vi "TCPIP_main.vi"() -> ()   [LabVIEW 2018]
uses:
  <vilib>/Utility/error.llb/DialogType.ctl
  TCPIP_main_global.vi
panel:
  in  "Write+Read 2":bool
  out "data out":string
  in  "stop":bool
  in  "Write+Read":bool
  in  "Write":bool
  # "Please run python first\n.exe or .py\npython is server"
  # "This is a template for\nsomeone who don't\nuse pythonnode or \nhave trouble to install \ntensorflow, you can \ntrigger python by tcpip"
  # "Rikcy"
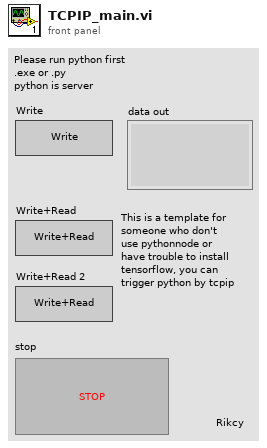
[diagram p1: front panel]
types:
  T1 = typedef "DialogType.ctl" = u16
  T2 = enum16{"Standard", "Buffered", "CRLF", "Immediate"}
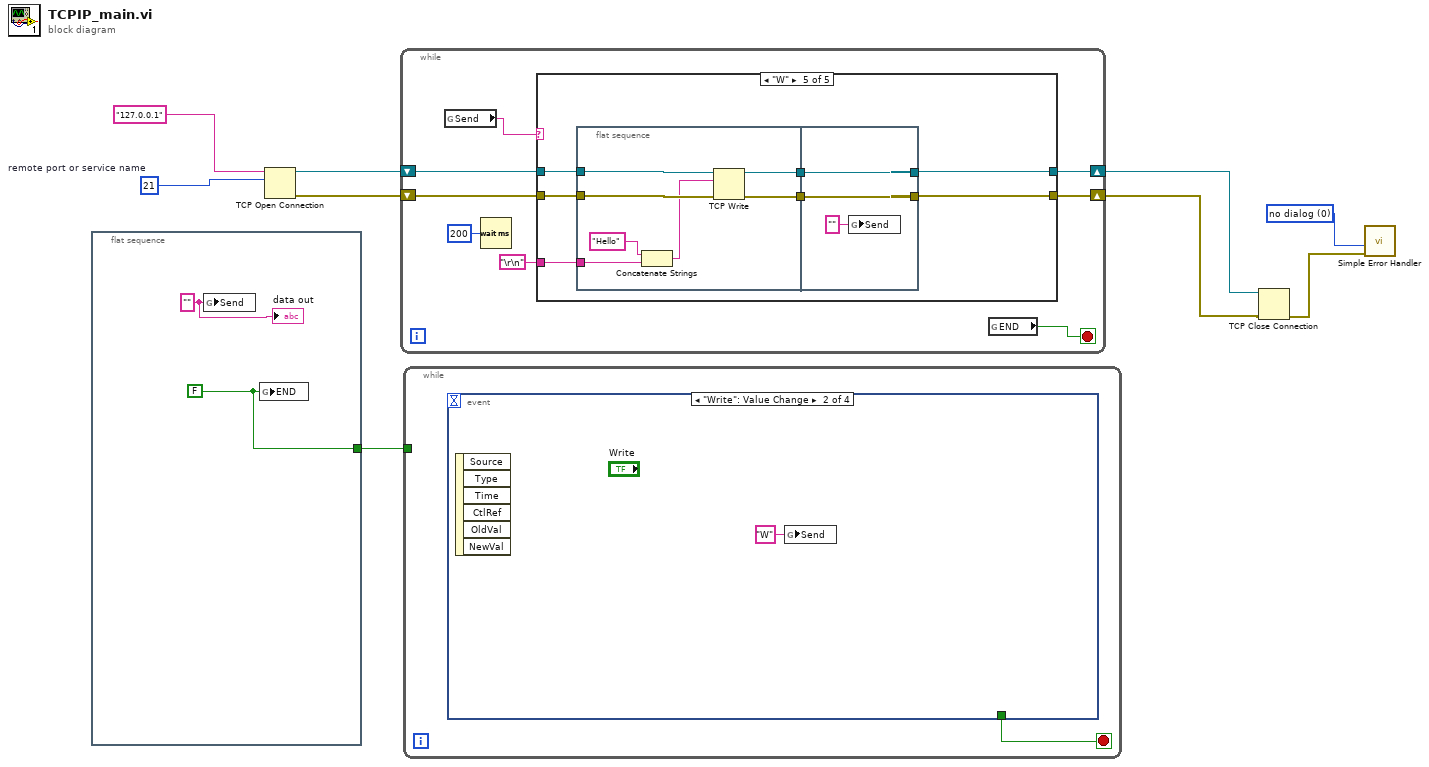
[diagram p0: block diagram]
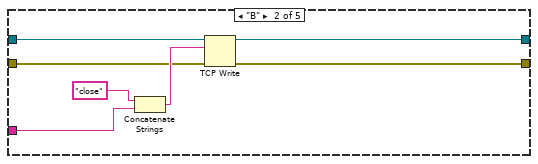
[diagram p3: hidden frame]
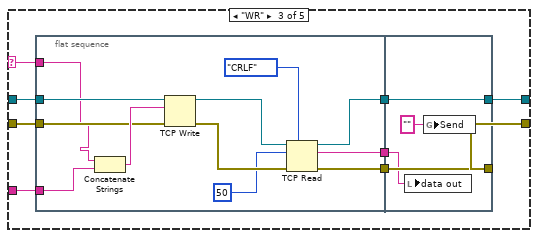
[diagram p4: hidden frame]
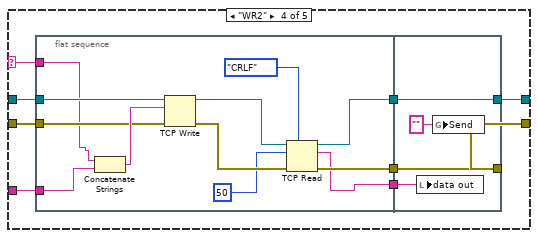
[diagram p5: hidden frame]
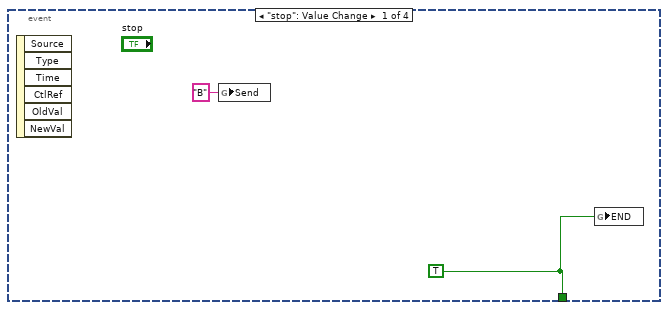
[diagram p6: hidden frame]
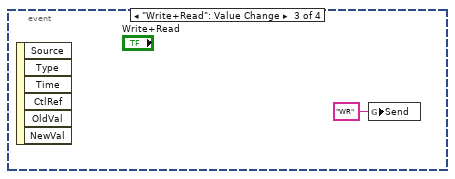
[diagram p7: hidden frame]
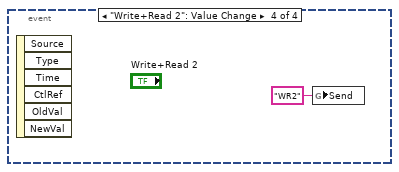
[diagram p8: hidden frame]
diagram:
  w1 = T1 0 items=["no dialog", "OK message", "continue or stop message", "OK message + warnings", "continue/stop + warnings"] ("type of dialog (OK msg:1)")
  w3 = u16 21  # remote port or service name
  n1 = flat-sequence {
    tunnel: [w11] -> w7
    frame #0 {
      w10 = "" ("Send")
      w11 = FALSE ("END")
      n2 = global write "TCPIP_main_global.vi" "Send"(w10) -> ()
      n3 = global write "TCPIP_main_global.vi" "END"(w11) -> ()
      "data out" <- w10
    }
  }
  n4 = TCP Open Connection(address="127.0.0.1", remote port or service name=w3) -> (connection ID=w9:refnum<k5>, error out=w8:errorcluster)  [unwired: 3 in]
  n5 = while {
    shift-right: [w14] -> w5
    shift-left: w9 -> [w19]
    shift-right: [w13] -> w4
    shift-left: w8 -> [w18]
    stop <- w17 stop-if-true
    n6 = global read "TCPIP_main_global.vi" "Send"() -> (w15:string)
    n7 = Wait (ms)(milliseconds to wait=u32 200) -> ()  [unwired: 1 out]
    n8 = case shown="\"W\"" w15 {
      selector: w15 -> [_ _ w29 w54 _]
      tunnel: w19 -> [w21 w28 w37 w62 w85]
      tunnel: w18 -> [w20 w22 w36 w61 w84]
      tunnel: [w21 w27 w35 w60 w83] -> w14
      tunnel: [w20 w26 w34 w59 w82] -> w13
      tunnel: "\r\n" -> [_ w24 w33 w58 w81]
      frame "", Default {
      }
      frame "B" {
        n9 = Concatenate Strings("close" ("Send"), w24) -> (w23:string)
        n10 = TCP Write(connection ID=w28, data in=w23, error in (no error)=w22) -> (connection ID out=w27:refnum<k5>, error out=w26:errorcluster)  [unwired: 1 in, 1 out]
      }
      frame "WR" {
        n11 = flat-sequence {
          tunnel: w37 -> [w49]
          tunnel: w36 -> [w47]
          tunnel: w33 -> [w42]
          tunnel: [w45] -> w32
          tunnel: [w44] -> w31
          tunnel: [w39] -> w30
          tunnel: w29 -> [w38]
          tunnel: [w52] -> w34
          tunnel: [w53] -> w35
          tunnel: w32 -> [w53]
          tunnel: w31 -> [w52]
          tunnel: w30 -> [w50]
          frame #0 {
            n12 = Concatenate Strings(w38, w42) -> (w48:string)
            n13 = TCP Write(connection ID=w49, data in=w48, error in (no error)=w47) -> (connection ID out=w46:refnum<k5>, error out=w43:errorcluster)  [unwired: 1 in, 1 out]
            n14 = TCP Read(connection ID=w46, bytes to read=50, error in (no error)=w43, 7:T2."CRLF" ("mode (standard)")) -> (connection ID out=w45:refnum<k5>, data out=w39:string, error out=w44:errorcluster)  [unwired: 1 in]
          }
          frame #1 {
            n15 = local write "data out"(w50) -> ()
            n16 = global write "TCPIP_main_global.vi" "Send"("" ("Send")) -> ()
          }
        }
      }
      frame "WR2" {
        n17 = flat-sequence {
          tunnel: w62 -> [w74]
          tunnel: w61 -> [w72]
          tunnel: w58 -> [w67]
          tunnel: [w70] -> w57
          tunnel: [w69] -> w56
          tunnel: [w64] -> w55
          tunnel: w54 -> [w63]
          tunnel: [w77] -> w59
          tunnel: [w78] -> w60
          tunnel: w57 -> [w78]
          tunnel: w56 -> [w77]
          tunnel: w55 -> [w75]
          frame #0 {
            n18 = Concatenate Strings(w63, w67) -> (w73:string)
            n19 = TCP Write(connection ID=w74, data in=w73, error in (no error)=w72) -> (connection ID out=w71:refnum<k5>, error out=w68:errorcluster)  [unwired: 1 in, 1 out]
            n20 = TCP Read(connection ID=w71, bytes to read=50, error in (no error)=w68, 7:T2."CRLF" ("mode (standard)")) -> (connection ID out=w70:refnum<k5>, data out=w64:string, error out=w69:errorcluster)  [unwired: 1 in]
          }
          frame #1 {
            n21 = local write "data out"(w75) -> ()
            n22 = global write "TCPIP_main_global.vi" "Send"("" ("Send")) -> ()
          }
        }
      }
      frame "W" {
        n23 = flat-sequence {
          tunnel: w85 -> [w92]
          tunnel: w84 -> [w91]
          tunnel: w81 -> [w87]
          tunnel: [w90] -> w80
          tunnel: [w89] -> w79
          tunnel: [w94] -> w82
          tunnel: [w95] -> w83
          tunnel: w80 -> [w95]
          tunnel: w79 -> [w94]
          frame #0 {
            n24 = Concatenate Strings("Hello" ("data in"), w87) -> (w86:string)
            n25 = TCP Write(connection ID=w92, data in=w86, error in (no error)=w91) -> (connection ID out=w90:refnum<k5>, error out=w89:errorcluster)  [unwired: 1 in, 1 out]
          }
          frame #1 {
            n26 = global write "TCPIP_main_global.vi" "Send"("" ("Send")) -> ()
          }
        }
      }
    }
    n27 = global read "TCPIP_main_global.vi" "END"() -> (w17:bool)
  }
  n28 = while {
    tunnel: w7 -> [_]
    stop <- w96 stop-if-true
    n29 = event shown="[1] \"Write\": Value Change" {
      selector: _ -> [_ _ _ _]
      dyn-events: _ -> [_ _ _ _]
      timeout: _ -> [_ _ _ _]
      tunnel: [w98 _ _ _] -> w96
      event "stop": Value Change {
        w98 = TRUE
        n30 = event-data() -> ()  [unwired: 1 in, 6 out]
        n31 = global write "TCPIP_main_global.vi" "Send"("B" ("Send")) -> ()
        n32 = global write "TCPIP_main_global.vi" "END"(w98) -> ()
      }
      event "Write": Value Change {
        n33 = event-data() -> ()  [unwired: 1 in, 6 out]
        n34 = global write "TCPIP_main_global.vi" "Send"("W" ("Send")) -> ()
      }
      event "Write+Read": Value Change {
        n35 = event-data() -> ()  [unwired: 1 in, 6 out]
        n36 = global write "TCPIP_main_global.vi" "Send"("WR" ("Send")) -> ()
      }
      event "Write+Read 2": Value Change {
        n37 = event-data() -> ()  [unwired: 1 in, 6 out]
        n38 = global write "TCPIP_main_global.vi" "Send"("WR2" ("Send")) -> ()
      }
    }
  }
  n39 = TCP Close Connection(connection ID=w5, error in (no error)=w4) -> (error out=w2:errorcluster)  [unwired: 1 in, 1 out]
  n40 = call <vilib>:"Simple Error Handler.vi"("type of dialog (OK msg:1)"=w1, "error in (no error)"=w2) -> ()  [unwired: 3 in, 5 out]
